vi "Remove Empty Space FromElements Return Warning.vi"(8 "error in (no error)":errorcluster, 10 "String Array In":string[](array[string])) -> (0 "error out":errorcluster, 2 "String Array Out":string[](array[string]))   [LabVIEW 2015, in "Case Manipulation.lvlib"]
uses:
  Case Manipulation.lvlib
  <vilib>/ErrorRing/Error Ring.xnode
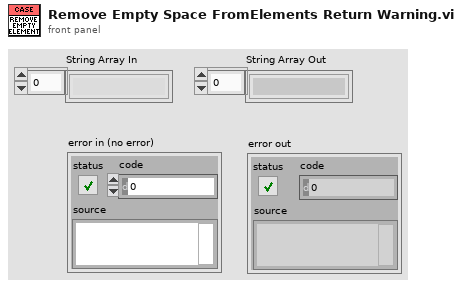
[diagram p1: front panel]
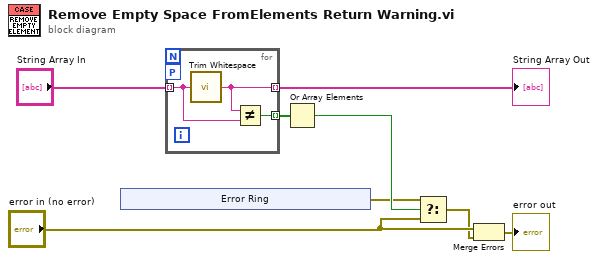
[diagram p0: block diagram]
diagram:
  n1 = xnode "Error Ring"() -> ("error out"=w5:errorcluster)
  n2 = for {
    tunnel: "String Array In" -> [w10] mode=indexing
    tunnel: [w11] -> w8 mode=indexing
    workers-P: _ -> [_]
    tunnel: [w9] -> w7 mode=indexing
    n3 = call <vilib>:"Trim Whitespace.vi"("string"=w10) -> ("trimmed string"=w11:string)  [unwired: 1 in]
    n4 = Not Equal?(x=w11, y=w10) -> (x != y?=w9:bool)
  }
  "String Array Out" <- w8
  n5 = Or Array Elements(Boolean array=w7) -> (logical OR=w6:bool)
  n6 = Select(t=w5, s=w6, f="error in (no error)") -> (s? t:f=w2:errorcluster)
  n7 = Merge Errors("error in (no error)", w2) -> (→"error out":errorcluster)
